vi "RSZVB Set Automatic Power Reduction State.vi"(8 "error in (no error)":errorcluster {"code" format="%.0x"}, 9 "Automatic Power Reduction (Off)":bool, 11 "VISA session":refnum<visa-resource-name>) -> (0 "error out":errorcluster {"code" format="%.0x"}, 3 "dup VISA session":refnum<visa-resource-name>)   [LabVIEW 2011]
doc: "This VI enables or disables automatic power reduction at all test ports while an automatic calibration using the\ncalibration unit R&S ZV-Zxx is active. \n\nRemote-control command(s):\nSYSTem:COMMunicate:RDEVice:AKAL:PREDuction[:STATe] ON | OFF"
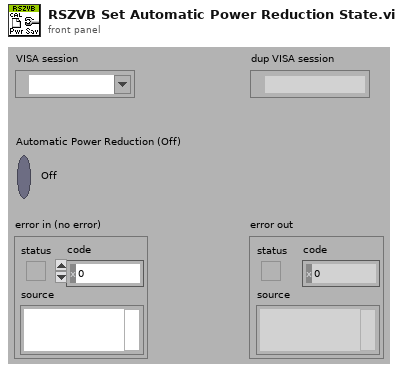
[diagram p1: front panel]
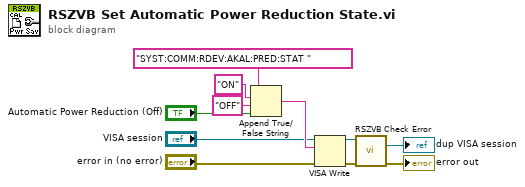
[diagram p0: block diagram]
diagram:
  n1 = Append True/False String(1:"Automatic Power Reduction (Off)", 2:"OFF" ("false string"), 3:"ON" ("true string"), 4:"SYST:COMM:RDEV:AKAL:PRED:STAT " ("string (\"\")")) -> (0:w6:string)
  n2 = VISA Write(VISA resource name="VISA session", write buffer=w6, error in (no error)="error in (no error)") -> (VISA resource name out=w8:refnum<visa-resource-name>, error out=w9:errorcluster)  [unwired: 1 out]
  n3 = call "RSZVB Check Error.vi"("error in (no error)"=w9, "VISA session"=w8) -> ("error out"=→"error out":errorcluster, "dup VISA session"=→"dup VISA session":refnum<visa-resource-name>)  [unwired: 8 in]
